vi "HGF_DSCEvent.appendData2Variant.vi"(0 "initData":variant, 5 "error in (no error)":errorcluster, 8 "HGF_Event (Monitor Event)":refnum<class "HGF_Event.lvclass">) -> (14 "dup initData":variant, 19 "error out":errorcluster)   [LabVIEW 2012, in "HGF_DSC.lvlib" / "HGF_DSCEvent.lvclass"]
uses:
  HGF_DSCEvent.lvclass
  HGF_BaseClasses/HGF_Event/HGF_Event.lvclass
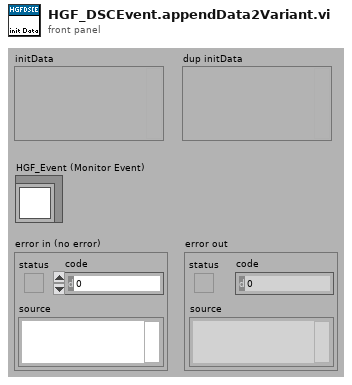
[diagram p1: front panel]
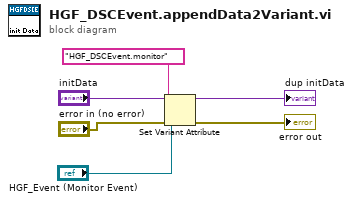
[diagram p0: block diagram]
diagram:
  n1 = Set Variant Attribute(Variant="initData", name="HGF_DSCEvent.monitor", value="HGF_Event (Monitor Event)", error in="error in (no error)") -> (Variant out=→"dup initData":variant, error out=→"error out":errorcluster)  [unwired: 1 out]
